vi "EncoderStart.vi"(0 "Device Info":T1={"Serial Number"=-1, "Channel"=0, "Port"=0}, 1 "Data Interval":i32=-1, 2 "Change Trigger":i32, 5 "Enabled":bool=TRUE, 7 "IO Mode":i32(ring)=1 items=["ENCODER_IO_MODE_PUSH_PULL"=1, "ENCODER_IO_MODE_LINE_DRIVER_2K2"=2, "ENCODER_IO_MODE_LINE_DRIVER_10K"=3, "ENCODER_IO_MODE_OPEN_COLLECTOR_2K2"=4, "ENCODER_IO_MODE_OPEN_COLLECTOR_10K"=5], 11 "error in (no error)":errorcluster, 12 "Connection":u16(ring) items=["No Preference", "Remote", "Local"], 13 "Timeout (mSec)":i32=5000) -> (4 "Phidget ID":u64, 6 "Serial Number Return":i32, 10 "Attached?":bool, 15 "error out":errorcluster)   [LabVIEW 2020, in "Phidget Encoder.lvlib"]
doc: "${Encoder:StartHeader}"
uses:
  <instrlib>/Phidgets/Phidget Encoder/Phidget Encoder.lvlib
  <instrlib>/Phidgets/Phidget Common/Phidget Common.lvlib
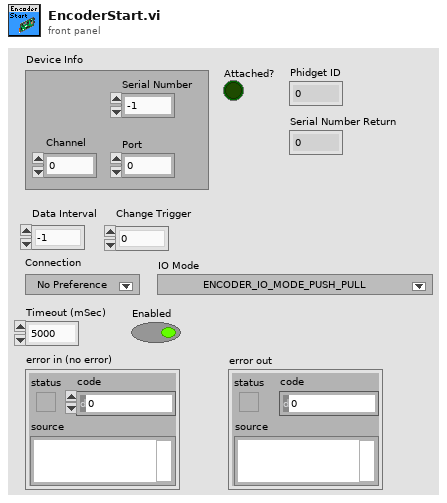
[diagram p1: front panel]
types:
  T1 = cluster{"Serial Number":i32, "Channel":i32, "Port":i32}
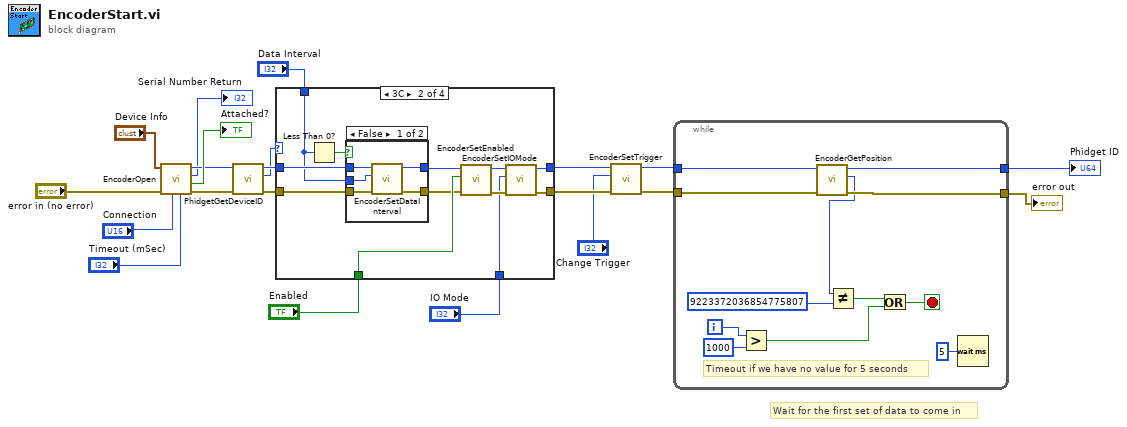
[diagram p0: block diagram]
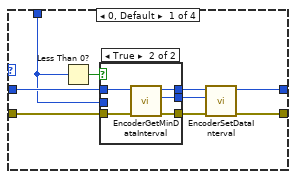
[diagram p2: hidden frame]
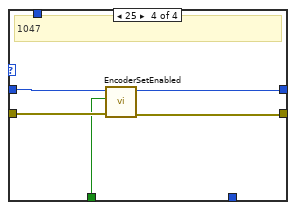
[diagram p6: hidden frame]
diagram:
  # "Wait for the first set of data to come in"
  n1 = call <instrlib>:"EncoderOpen.vi"("Timeout (mSec)"="Timeout (mSec)", "Connection"="Connection", "error in"="error in (no error)", "Device Info"="Device Info") -> ("error out"=w18:errorcluster, "Attached?"=→"Attached?":bool, "Serial Number Return"=→"Serial Number Return":i32, "Phidget ID"=w17:u64)  [unwired: 4 in]
  n2 = call <instrlib>:"PhidgetGetDeviceID.vi"("error in (no error)"=w18, "Device In"=w17) -> ("error out"=w15:errorcluster, "Devie IDs"=w14:u32, "Device Out"=w16:u64)  [unwired: 6 in]
  n3 = case shown="3C" w14 {
    tunnel: w15 -> [w27 w49 w59 w63]
    tunnel: [w30 w42 w59 w62] -> w10
    tunnel: w16 -> [w26 w48 w58 w64]
    tunnel: [w29 w43 w58 w61] -> w11
    tunnel: "Data Interval" -> [w25 w47 _ _]
    tunnel: "Enabled" -> [_ w46 _ w60]
    tunnel: "IO Mode" -> [_ w41 _ _]
    frame 0, Default {
      n4 = Less Than 0?(x=w25) -> (x < 0?=w28:bool)
      n5 = case shown="True" w28 {
        tunnel: w26 -> [w32 w38]
        tunnel: w27 -> [w31 w37]
        tunnel: [w32 w36] -> w23
        tunnel: [w31 w35] -> w24
        tunnel: [w33 w34] -> w22
        tunnel: w25 -> [w33 _]
        frame False {
        }
        frame True {
          n6 = call <instrlib>:"EncoderGetMinDataInterval.vi"("error in (no error)"=w37, "Device In"=w38) -> ("error out"=w35:errorcluster, "Min Data Interval"=w34:i32, "Device Out"=w36:u64)  [unwired: 6 in]
        }
      }
      n7 = call <instrlib>:"EncoderSetDataInterval.vi"("error in (no error)"=w24, "Interval"=w22, "Device In"=w23) -> ("error out"=w30:errorcluster, "Device Out"=w29:u64)  [unwired: 6 in]
    }
    frame 60 {
      n8 = Less Than 0?(x=w47) -> (x < 0?=w50:bool)
      n9 = case shown="False" w50 {
        tunnel: w48 -> [w54 w57]
        tunnel: w49 -> [w55 w56]
        tunnel: [w53 w57] -> w39
        tunnel: [w52 w56] -> w40
        tunnel: w47 -> [w51 _]
        frame False {
          n10 = call <instrlib>:"EncoderSetDataInterval.vi"("error in (no error)"=w55, "Interval"=w51, "Device In"=w54) -> ("error out"=w52:errorcluster, "Device Out"=w53:u64)  [unwired: 6 in]
        }
        frame True {
        }
      }
      n11 = call <instrlib>:"EncoderSetEnabled.vi"("error in (no error)"=w40, "Enabled"=w46, "Device In"=w39) -> ("error out"=w45:errorcluster, "Device Out"=w44:u64)  [unwired: 6 in]
      n12 = call <instrlib>:"EncoderSetIOMode.vi"("error in (no error)"=w45, "IO Mode"=w41, "Device In"=w44) -> ("error out"=w42:errorcluster, "Device Out"=w43:u64)  [unwired: 6 in]
    }
    frame 29, 34, 42 {
      # "Do not set\ndata interval on\ndevices that\ndon't support it"
      # "1052, 1057, 1065"
    }
    frame 25 {
      # "1047"
      n13 = call <instrlib>:"EncoderSetEnabled.vi"("error in (no error)"=w63, "Enabled"=w60, "Device In"=w64) -> ("error out"=w62:errorcluster, "Device Out"=w61:u64)  [unwired: 6 in]
    }
  }
  n14 = call <instrlib>:"EncoderSetTrigger.vi"("error in (no error)"=w10, "Trigger"="Change Trigger", "Device In"=w11) -> ("error out"=w3:errorcluster, "Device Out"=w4:u64)  [unwired: 6 in]
  n15 = while {
    tunnel: w4 -> [w74]
    tunnel: w3 -> [w73]
    tunnel: [w71] -> w13
    tunnel: [w72] -> w20
    i -> [w69]
    stop <- w66 stop-if-true
    # "Timeout if we have no value for 5 seconds"
    n16 = Greater?(x=w69, y=1000) -> (0:w67:bool)
    n17 = call <instrlib>:"EncoderGetPosition.vi"("error in (no error)"=w73, "Device In"=w74) -> ("error out"=w72:errorcluster, "Position"=w65:i64, "Device Out"=w71:u64)  [unwired: 6 in]
    n18 = Not Equal?(x=w65, y=i64 9223372036854775807) -> (x != y?=w68:bool)
    n19 = Or(x=w68, y=w67) -> (x .or. y?=w66:bool)
    n20 = Wait (ms)(milliseconds to wait=u32 5) -> ()  [unwired: 1 out]
  }
  "error out" <- w20
  "Phidget ID" <- w13
